vi "globalSetUp.vi"(8 "error in":errorcluster, 11 "Single Core Complex Loopback in":refnum<class "Single Core Complex Loopback.lvclass">) -> (0 "error out":errorcluster, 3 "Single Core Complex Loopback out":refnum<class "Single Core Complex Loopback.lvclass">)   [LabVIEW 2020, in "Single Core Complex Loopback.lvclass"]
uses:
  Single Core Complex Loopback.lvclass
  niveristand-custom-device-testing-tools/VeriStandTestUtilities/VeriStandTestUtilities.lvlib
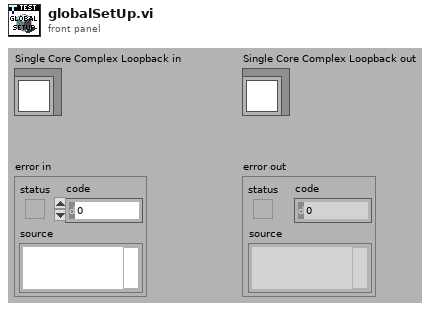
[diagram p1: front panel]
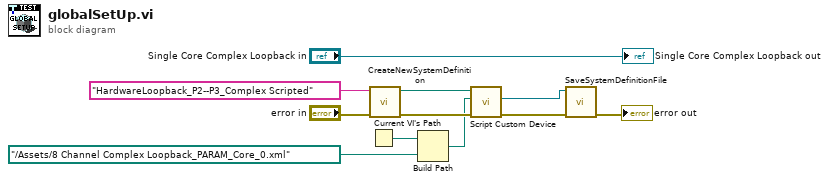
[diagram p0: block diagram]
diagram:
  n1 = Current VI's Path() -> (path=w9:path)
  n2 = call "CreateNewSystemDefinition.vi"("error in"="error in", "System Definition Name"="HardwareLoopback_P2--P3_Complex Scripted" ("Channel")) -> ("error out"=w11:errorcluster, "System Definition Path"=w10:path)  [unwired: 8 in]
  n3 = Build Path(base path=w9, name or relative path=path "../Assets/8 Channel Complex Loopback_PARAM_Core_0.xml" ("Hardware File Path")) -> (appended path=w1:path)
  n4 = call "Script Custom Device.vi"("error in"=w11, "Parameter File Path"=w1, "System Definition File Path In"=w10) -> ("error out"=w6:errorcluster, "System Definition Reference"=w2:refnum<k24>)  [unwired: 5 in, 2 out]
  n5 = call "SaveSystemDefinitionFile.vi"("error in (no error)"=w6, "System Definition Reference in"=w2) -> ("error out"=→"error out":errorcluster)  [unwired: 8 in, 1 out]
  "Single Core Complex Loopback out" <- "Single Core Complex Loopback in"
